vi "Launch Asynchronously.vi"(8 "error in (no error)":errorcluster, 11 "Runnable in":refnum<class "Runnable.lvclass">) -> (0 "error out":errorcluster)   [LabVIEW 2020, in "Parallell Test Runner.lvclass"]
uses:
  Parallell Test Runner.lvclass
  Run/Runnable.lvclass
  Execute.vi
  Parallell Test Runner.lvclass/Parallell Test Runner.ctl
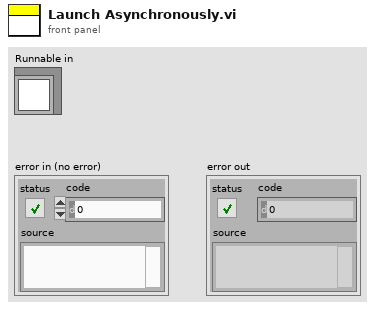
[diagram p1: front panel]
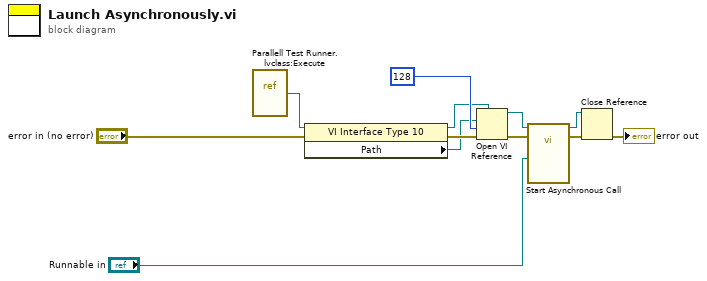
[diagram p0: block diagram]
diagram:
  n1 = vi-ref "Parallell Test Runner.lvclass:Execute.vi"() -> (w1:refnum<vi>)
  n2 = property class="VI Interface Type 10"(reference=w1, error in="error in (no error)") -> (reference out=w3:refnum<vi>, error out=w4:errorcluster, "Path"=w2:path)
  n3 = Open VI Reference(type specifier VI Refnum (for type only)=w3, vi path=w2, options=128, error in (no error)=w4) -> (vi reference=w5:refnum<vi>, error out=w6:errorcluster)  [unwired: 2 in]
  n4 = call-by-ref "Start Asynchronous Call"(reference=w5, error in=w6, "Test Runner V2 in"="Runnable in") -> (reference out=w7:refnum<vi>, error out=w8:errorcluster)  [unwired: 11 in]
  n5 = Close Reference(reference=w7, error in (no error)=w8) -> (error out=→"error out":errorcluster)
